vi "Виртуальный прибор курсовой работы.vi"() -> ()   [LabVIEW 2020]
uses:
  <vilib>/Instr/_visa.llb/VISA Configure Serial Port (Instr).vi
panel:
  in  "stop":bool
  in  "baud rate (9600)":u32=9600
  in  "Boolean":bool
  in  "VISA resource name":refnum<visa-resource-name>
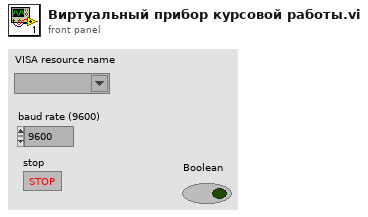
[diagram p1: front panel]
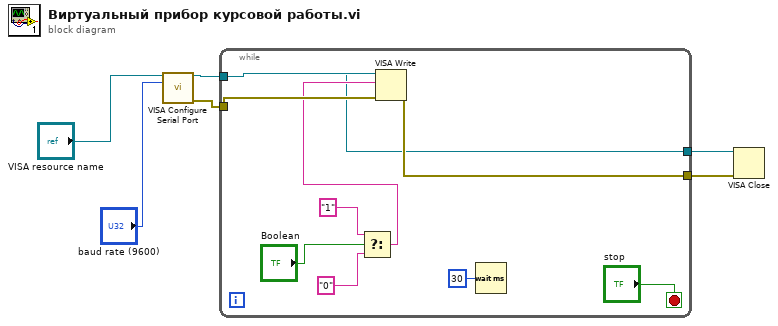
[diagram p0: block diagram]
diagram:
  n1 = call-poly "VISA Configure Serial Port"("VISA resource name"="VISA resource name", "baud rate (9600)"="baud rate (9600)") -> ("VISA resource name out"=w5:refnum<visa-resource-name>, "error out"=w4:errorcluster)  [unwired: 12 in]
  n2 = while {
    tunnel: w5 -> [w16]
    tunnel: w4 -> [w15]
    tunnel: [w7] -> w3
    tunnel: [w14] -> w2
    stop <- "stop" stop-if-true
    n3 = Select(t="1", s="Boolean", f="0") -> (s? t:f=w10:string)
    n4 = VISA Write(VISA resource name=w16, write buffer=w10, error in (no error)=w15) -> (VISA resource name out=w7:refnum<visa-resource-name>, error out=w14:errorcluster)  [unwired: 1 out]
    n5 = Wait (ms)(milliseconds to wait=u32 30) -> ()  [unwired: 1 out]
  }
  n6 = VISA Close(VISA resource name=w3, error in (no error)=w2) -> ()  [unwired: 1 out]
